vi "helper1.vi"(8 "error in (no error)":errorcluster, 11 "y":string="Sub Panel") -> (0 "error out":errorcluster, 3 "Array":string[](array[string]))   [LabVIEW 2021]
panel:
  out "Array 2":string[](array[string])
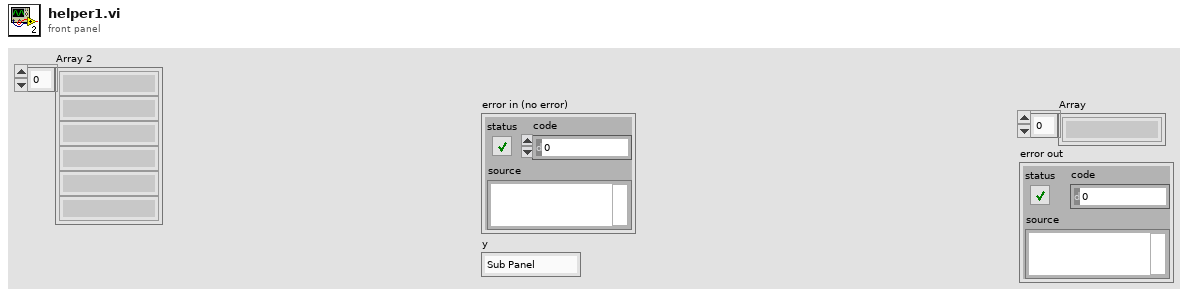
[diagram p1: front panel]
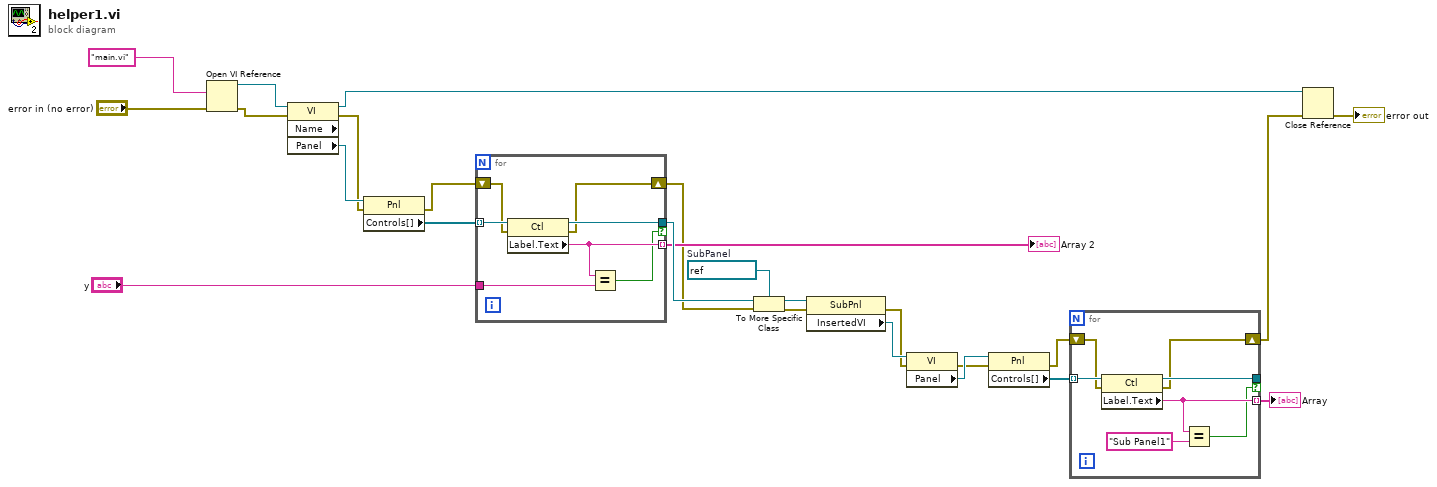
[diagram p0: block diagram]
diagram:
  w21 = refnum<vi> refnum  # SubPanel
  n1 = Open VI Reference(vi path="main.vi" ("machine name (\"\":  open local reference)"), error in (no error)="error in (no error)") -> (vi reference=w15:refnum<vi>, error out=w14:errorcluster)  [unwired: 4 in]
  n2 = property class="VI" props=["Name", "Panel"](reference=w15, error in=w14) -> (reference out=w1:refnum<vi>, error out=w9:errorcluster, "Panel"=w16:refnum<vi>)  [unwired: 1 out]
  n3 = property class="Pnl"(reference=w16, error in=w9) -> (error out=w8:errorcluster, "Controls[]"=w17:refnum<vi>[])  [unwired: 1 out]
  n4 = for {
    tunnel: w17 -> [w32] mode=indexing
    tunnel: [w31] -> w18 mode=indexing
    shift-right: [w26] -> w7
    shift-left: w8 -> [w27]
    tunnel: [w30] -> w19 if=w29
    tunnel: "y" -> [w28]
    n5 = property class="Ctl"(reference=w32, error in=w27) -> (reference out=w30:refnum<vi>, error out=w26:errorcluster, "Label.Text"=w31:string)
    n6 = Equal?(x=w31, y=w28) -> (x = y?=w29:bool)
  }
  "Array 2" <- w18
  n7 = To More Specific Class(target class=w21, reference=w19, error in=w7) -> (specific class reference=w20:refnum<vi>, error out=w6:errorcluster)
  n8 = property class="SubPnl"(reference=w20, error in=w6) -> (error out=w5:errorcluster, "InsertedVI"=w24:refnum<vi>)  [unwired: 1 out]
  n9 = property class="VI"(reference=w24, error in=w5) -> (error out=w23:errorcluster, "Panel"=w25:refnum<vi>)  [unwired: 1 out]
  n10 = property class="Pnl"(reference=w25, error in=w23) -> (error out=w4:errorcluster, "Controls[]"=w22:refnum<vi>[])  [unwired: 1 out]
  n11 = for {
    tunnel: w22 -> [w39] mode=indexing
    tunnel: [w38] -> w11 mode=indexing
    shift-right: [w33] -> w3
    shift-left: w4 -> [w34]
    tunnel: [w36] -> _ if=w35
    n12 = property class="Ctl"(reference=w39, error in=w34) -> (reference out=w36:refnum<vi>, error out=w33:errorcluster, "Label.Text"=w38:string)
    n13 = Equal?(x=w38, y="Sub Panel1") -> (x = y?=w35:bool)
  }
  "Array" <- w11
  n14 = Close Reference(reference=w1, error in (no error)=w3) -> (error out=→"error out":errorcluster)
